vi "Untitled 2.vi"() -> ()   [LabVIEW 2020]
uses:
  <vilib>/httpClient/PUTBuffer.vi
  <vilib>/httpClient/LabVIEWHTTPClient.lvlib
panel:
  in  "Hora":string
  in  "Data":string
  in  "Accionamiento [mA]":dbl(knob) scale=0.0..10.0
  in  "Rele":bool
  in  "stop 2":bool
  out "error out":errorcluster {"code" format="%f"}
  out "body":string
  out "headers":string
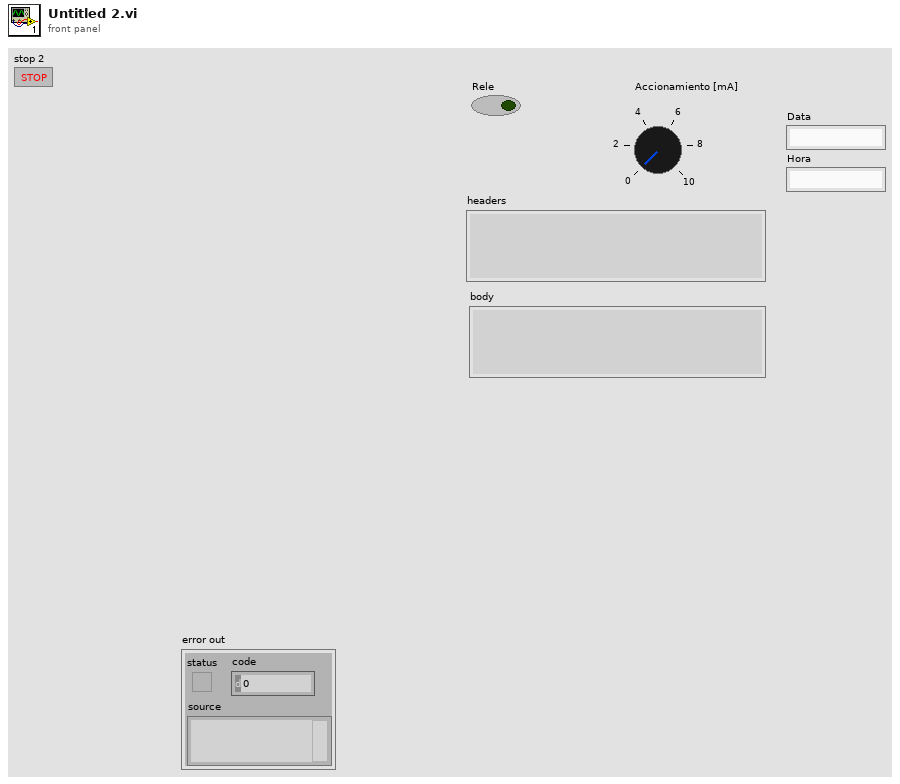
[diagram p1: front panel]
types:
  T1 = cluster{"Accionamiento":dbl, "Data":string, "Hora":string, "Rele":bool}
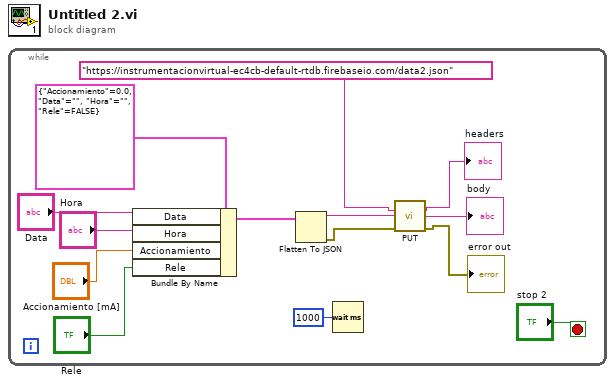
[diagram p0: block diagram]
diagram:
  n1 = while {
    stop <- "stop 2" stop-if-true
    n2 = Bundle By Name(cluster=T1 {"Accionamiento"=0.0, "Data"="", "Hora"="", "Rele"=FALSE}, "Data"="Data", "Hora"="Hora", "Accionamiento"="Accionamiento [mA]", "Rele"="Rele") -> (w12:T1)
    n3 = Flatten To JSON(anything=w12) -> (JSON string=w3:string, 11:w4:errorcluster)  [unwired: 2 in]
    n4 = Wait (ms)(milliseconds to wait=u32 1000) -> ()  [unwired: 1 out]
    n5 = call-poly <vilib>:"PUT.vi"("url"="https://instrumentacionvirtual-ec4cb-default-rtdb.firebaseio.com/data2.json", "buffer"=w3, "error in (no error)"=w4) -> ("headers"=→"headers":string, "body"=→"body":string, "error out"=→"error out":errorcluster)  [unwired: 9 in, 1 out]
  }
